vi "Cannon Process.vi"(0 "error in":errorcluster) -> ()   [LabVIEW 2012]
uses:
  Cannon Global Data.vi
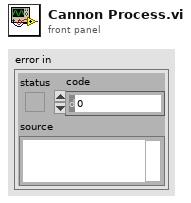
[diagram p1: front panel]
types:
  T1 = cluster{"RPM":dbl, "Trigger":bool, "Angle Axis":dbl, "Angle":dbl, "Throttle":dbl, "Slow Angle Change?":bool, "Angle Change?":bool}
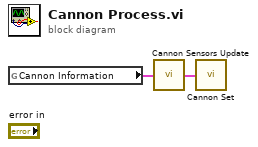
[diagram p0: block diagram]
diagram:
  n1 = global read "Cannon Global Data.vi" "Cannon Information"() -> (w2:T1)
  n2 = call "Cannon Sensors Update.vi"("Cannon Information"=w2) -> ("Cannon Information out"=w1:T1)
  n3 = call "Cannon Set.vi"("Cannon Information"=w1) -> ()
